vi "CW Creator.vi"(10 "Plaintext to CW Map":map{string, bool[]}(c390), 11 "Plaintext Array":string[](array[string])) -> ()   [LabVIEW 2026]
panel:
  out "CW Array":bool[][](array[boolean])
  out "error out":errorcluster
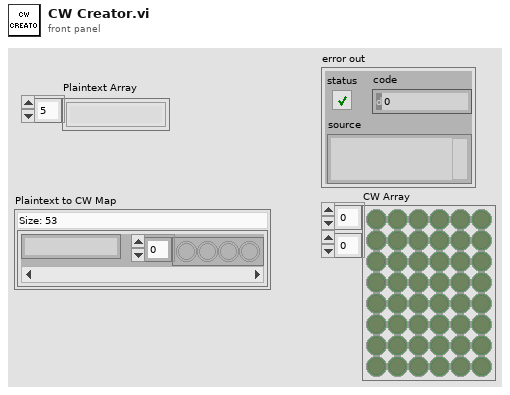
[diagram p1: front panel]
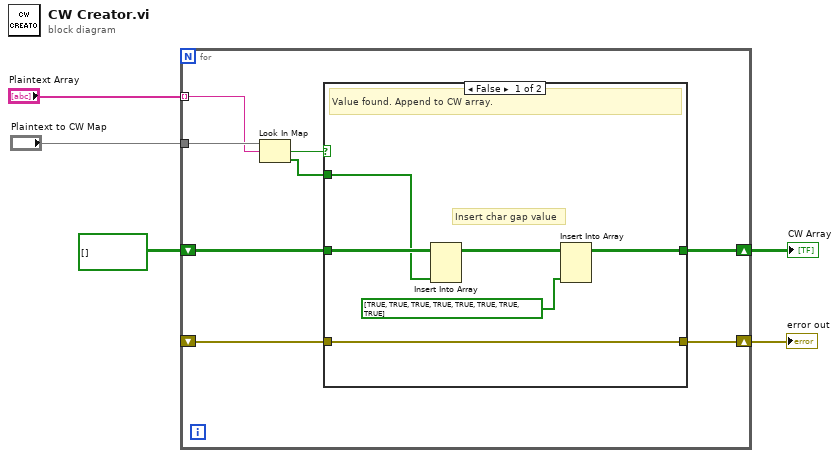
[diagram p0: block diagram]
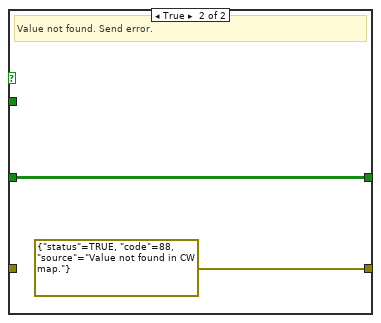
[diagram p2: hidden frame]
diagram:
  n1 = for {
    tunnel: "Plaintext Array" -> [w12] mode=indexing
    tunnel: "Plaintext to CW Map" -> [w13]
    shift-right: [w10] -> w2
    shift-left: _ -> [w9]
    shift-right: [w6] -> w1
    shift-left: bool[][] [] -> [w7]
    n2 = Look In Map(map=w13, key=w12) -> (key not found?=w11:bool, value=w8:bool[])  [unwired: 1 in]
    n3 = case shown="False" w11 {
      tunnel: [w19 errorcluster {"status"=TRUE, "code"=88, "source"="Value not found in CW map."} ("error constant")] -> w10
      tunnel: w9 -> [w19 _]
      tunnel: w8 -> [w17 _]
      tunnel: w7 -> [w18 w20]
      tunnel: [w14 w20] -> w6
      frame False {
        # "Insert char gap value"
        # "Value found. Append to CW array."
        n4 = Insert Into Array(array=w18, new element=w17) -> (w16:bool[][])  [unwired: 2 in]
        n5 = Insert Into Array(array=w16, new element=bool[] [TRUE, TRUE, TRUE, TRUE, TRUE, TRUE, TRUE, TRUE] ("new element/subarray")) -> (w14:bool[][])  [unwired: 2 in]
      }
      frame True {
        # "Value not found. Send error."
      }
    }
  }
  "error out" <- w2
  "CW Array" <- w1
